vi "Generate Maze.vi"(8 "error in (no error)":errorcluster, 9 "Height":i32, 10 "Width":i32, 11 "MazeGen in":refnum<class "MazeGen.lvclass">) -> (0 "error out":errorcluster, 2 "Maze":refnum<class "Maze.lvclass">, 3 "MazeGen out":refnum<class "MazeGen.lvclass">)   [LabVIEW 2020, in "Maze.lvlib" / "MazeGen.lvclass"]
uses:
  MazeGen.lvclass
  Maze/Maze.lvclass
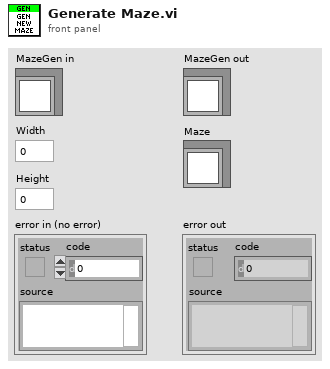
[diagram p1: front panel]
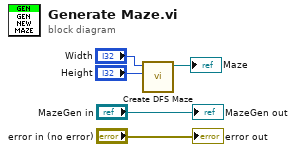
[diagram p0: block diagram]
diagram:
  n1 = call "Create DFS Maze.vi"("Height"="Height", "Width"="Width") -> ("Maze"=→"Maze":refnum<class "Maze.lvclass">)  [unwired: 9 in]
  "error out" <- "error in (no error)"
  "MazeGen out" <- "MazeGen in"
